vi "Try Send Message.vi"(8 "error in (no error)":errorcluster, 11 "OBS in":refnum<class "OBS.lvclass">) -> (0 "error out":errorcluster, 3 "OBS out":refnum<class "OBS.lvclass">)   [LabVIEW 2020, in "obs-websocket.lvlib" / "OBS.lvclass"]
uses:
  OBS.lvclass
  OBS.lvclass/OBS.ctl
  Request/Request.lvclass
  C:/dev/lv20CE/relink/lv-obs-websocket/obs-websocket/Client Message/Client Message.lvclass
  <vilib>/MediaMongrels Ltd/WebSockets/WebSockets/WebSocket Client/WebSocket Client.lvclass
  obs-websocket.lvlib
  Client Message/Client Message.lvclass
  lv-promises/Promises/Promise/Promise.lvclass
  C:/dev/lv20CE/relink/lv-obs-websocket/obs-websocket/Message/Message.lvclass
  C:/dev/lv20CE/relink/lv-obs-websocket/obs-websocket/Request/Request.lvclass
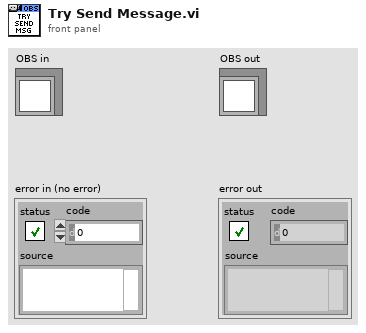
[diagram p1: front panel]
types:
  T1 = typedef "obs-websocket.lvlib/OBS.lvclass/Client Message.ctl" = cluster{"Message":refnum<class "Client Message.lvclass">, "Promise":refnum<class "Promise.lvclass">}
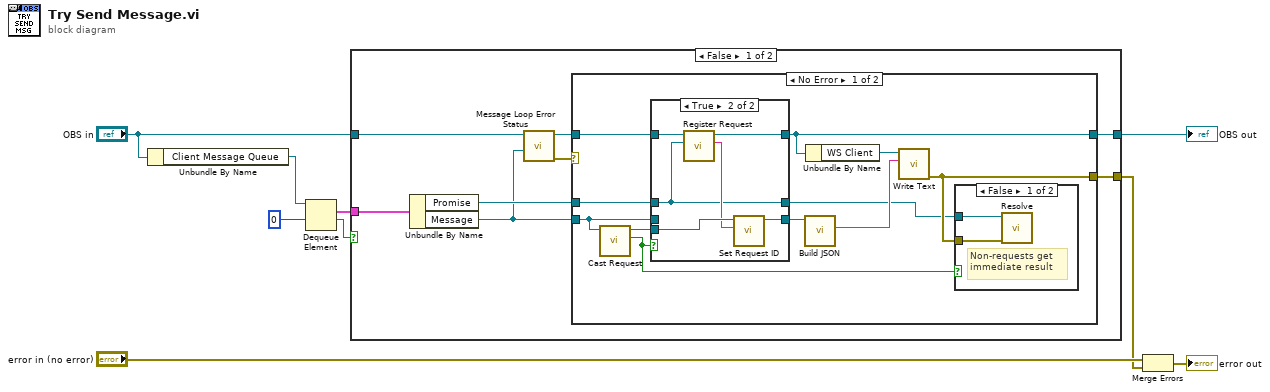
[diagram p0: block diagram]
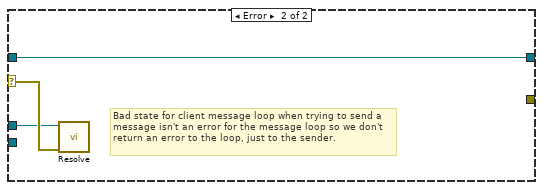
[diagram p4: hidden frame]
diagram:
  n1 = Unbundle By Name("OBS in") -> ("Client Message Queue"=w1:refnum<queue>)
  n2 = Dequeue Element(queue=w1, timeout in ms (-1)=0) -> (element=w6:T1, timed out?=w7:bool)  [unwired: 1 in, 2 out]
  n3 = case shown="False" w7 {
    tunnel: w6 -> [w10 _]
    tunnel: "OBS in" -> [w11 w43]
    tunnel: [w14 w43] -> w4
    tunnel: [w13 _] -> w2
    frame False {
      n4 = Unbundle By Name(w10) -> ("Promise"=w15:refnum<class "Promise.lvclass">, "Message"=w12:refnum<class "Client Message.lvclass">)
      n5 = call "Message Loop Error Status.vi"("Message"=w12, "OBS in"=w11) -> ("error out"=w17:errorcluster, "OBS out"=w16:refnum<class "OBS.lvclass">)  [unwired: 8 in]
      n6 = case shown="No Error" w17 {
        selector: w17 -> [_ w42]
        tunnel: w16 -> [w27 w41]
        tunnel: w15 -> [w25 w40]
        tunnel: [w21 w41] -> w14
        tunnel: [w28 _] -> w13
        tunnel: w12 -> [w18 _]
        frame No Error {
          n7 = call "Cast Request.vi"("Client Message"=w18) -> ("Is Request?"=w19:bool, "Request"=w26:refnum<class "Request.lvclass">)  [unwired: 9 in]
          n8 = case shown="True" w19 {
            tunnel: w27 -> [w33 w39]
            tunnel: w26 -> [_ w38]
            tunnel: w25 -> [w32 w34]
            tunnel: [w33 w36] -> w21
            tunnel: [w31 w35] -> w24
            tunnel: [w32 w34] -> w20
            tunnel: w18 -> [w31 _]
            frame False {
            }
            frame True {
              n9 = call "Register Request.vi"("Promise"=w34, "OBS in"=w39) -> ("Request ID"=w37:string, "OBS out"=w36:refnum<class "OBS.lvclass">)  [unwired: 7 in, 1 out]
              n10 = call "Set Request ID.vi"("Request ID"=w37, "Request in"=w38) -> ("Request out"=w35:refnum<class "Request.lvclass">)  [unwired: 8 in, 1 out]
            }
          }
          n11 = call "Build JSON.vi"("Client Message in"=w24) -> ("JSON"=w22:string)  [unwired: 8 in, 2 out]
          n12 = Unbundle By Name(w21) -> ("WS Client"=w23:refnum<class "WebSocket Client.lvclass">)
          n13 = call-dynamic "Write Text.vi"("String Data"=w22, "WebSocket in"=w23) -> ("error out"=w28:errorcluster)  [unwired: 8 in, 1 out]
          n14 = case shown="False" w19 {
            tunnel: w20 -> [w30 _]
            tunnel: w28 -> [w29 _]
            frame False {
              # "Non-requests get immediate result"
              n15 = call "Resolve.vi"("error in (no error)"=w29, "Promise in"=w30) -> ()  [unwired: 8 in, 2 out]
            }
            frame True {
              # "Requests will get response returned when read back from server."
            }
          }
        }
        frame Error {
          # "Bad state for client message loop when trying to send a message isn't an error for the message loop so we don't return an error to the loop, just to the sender."
          n16 = call "Resolve.vi"("error in (no error)"=w42, "Promise in"=w40) -> ()  [unwired: 8 in, 2 out]
        }
      }
    }
    frame True {
    }
  }
  "OBS out" <- w4
  n17 = Merge Errors("error in (no error)", w2) -> (→"error out":errorcluster)
